vi "test write read channel.vi"() -> ()   [LabVIEW 2013]
doc: "This VI is an example of how to use subVIs from the BNC 500 series driver to programmatically configure multiple channels and the system timer (To). This VI initializes the pulse generator, gets the number of channels in the unit, configures individual channel(s), configures the system timer (To), initiate pulse generation, and then closes communications with the pulse generator. By default the VI DOES NOT stop pulse generation when exiting!!! Not all trigger and gate features are supported by all models covered by this driver. Selection of an unsupported function will generate a software error and the command is not sent to the hardware.\n\n\nNotes:\n1) The pulse generator keypad is returned to \"Local\" mode when this VI terminates in order to restore manual control to the user.\n2) VISA Version 3.3 or higher must be installed to use this instrument driver."
uses:
  <instrlib>/Berkeley Nucleonics 500 Series/Examples/Support/System Parameters.ctl
  <instrlib>/Berkeley Nucleonics 500 Series/Examples/Support/Channel Parameters.ctl
  <instrlib>/Berkeley Nucleonics 500 Series/Berkeley Nucleonics 500 Series.lvlib
panel:
  in  "read back":bool
  in  "Channel Parameters 2":T1={"Channel"=1, "Chan State"=TRUE, "Chan Sync Source"=0, "Chan Gate Logic"=enum."Disabled", "Chan Mode"=enum."Normal", "Chan Wait #"=40, "Chan Delay"=0.04, "Chan Width"=0.04, "Chan Burst #"=40, "Chan DC On"=40, "Chan DC Off"=40, "Chan Polarity"=FALSE, "Chan MUX Value"=-1, "Chan Level Out"=enum."Adjustable", "Chan Lev Adjust"=0.0, "Chan Gate Mode"=enum."Disabled"} {"Chan Sync Source" items=["System (To)", "Channel A", "Channel B", "Channel C", "Channel D", "Channel E", "Channel F", "Channel G", "Channel H"]; "Chan Width" format="%.3p"; "Chan Delay" format="%.3p"; "Chan Lev Adjust" format="%.3p"; "Channel" items=["Channel A"=1, "Channel B"=2, "Channel C"=3, "Channel D"=4, "Channel E"=5, "Channel F"=6, "Channel G"=7, "Channel H"=8]}
  out "Chan Parameters":T1={"Channel"=1, "Chan State"=TRUE, "Chan Sync Source"=0, "Chan Gate Logic"=enum."Disabled", "Chan Mode"=enum."Normal", "Chan Wait #"=-1, "Chan Delay"=nan, "Chan Width"=nan, "Chan Burst #"=-1, "Chan DC On"=-1, "Chan DC Off"=-1, "Chan Polarity"=FALSE, "Chan MUX Value"=-1, "Chan Level Out"=enum."TTL", "Chan Lev Adjust"=0.0, "Chan Gate Mode"=enum."Disabled"} {"Chan Sync Source" items=["System (To)", "Channel A", "Channel B", "Channel C", "Channel D", "Channel E", "Channel F", "Channel G", "Channel H"]; "Chan Width" format="%.3p"; "Chan Delay" format="%.3p"; "Chan Lev Adjust" format="%.3p"; "Channel" items=["Channel A"=1, "Channel B"=2, "Channel C"=3, "Channel D"=4, "Channel E"=5, "Channel F"=6, "Channel G"=7, "Channel H"=8]}
  out "System Parameters":T2={"Sys Period"=0.1, "Sys Mode"=enum."Normal", "Sys Burst #"=10, "Sys DC On"=10, "Sys DC Off"=10, "Sys State"=TRUE, "Sys Gate"=TRUE, "Sys Trig Edge"=TRUE, "Sys Ext Mode"=enum."Disabled", "Sys Trig Lev"=2.5, "Sys Gate Lev "=2.5, "Sys Gate Mode"=enum."Disabled"} {"Sys Gate Lev" format="%.4p"; "Sys Trig Lev" format="%.4p"; "Sys Period" format="%.6p"}
  in  "VISA resource":refnum<visa-resource-name>="COM1"
  in  "System Paramaters":T2={"Sys Period"=0.1, "Sys Mode"=enum."Normal", "Sys Burst #"=0, "Sys DC On"=10, "Sys DC Off"=20, "Sys State"=TRUE, "Sys Gate"=TRUE, "Sys Trig Edge"=TRUE, "Sys Ext Mode"=enum."Disabled", "Sys Trig Lev"=2.5, "Sys Gate Lev "=2.5, "Sys Gate Mode"=enum."Disabled"} {"Sys Gate Lev" format="%.4p"; "Sys Trig Lev" format="%.4p"; "Sys Period" format="%.6p"}
  # "500 Series\nPulse Generator\nExample Program"
  # "Notes:\n1.  The channel parameters \"Burst #\", \"DC On\", \"DC Off\", and \"Adjustable\" are only updated when operating in the corresponding mode.\n2.  The system parameters  \"Burst #\", \"DC On\", \"DC Off\", and \"Trig Level\"` are only updated when operating in the corresponding mode."
  # "Input"
  # "Normal\nSingle\nBurst"
  # "Burst"
  # "Duty Cycle"
  # "Output"
  # "Input"
  # "Normal\nSingle\nBurst"
  # "Burst"
  # "Duty Cycle"
  # "Output"
  # "Input"
  # "Triggered"
  # "Gated"
  # "Mode"
  # "Burst"
  # "Duty\nCycle"
  # "Input"
  # "Triggered"
  # "Gated"
  # "Mode"
  # "Burst"
  # "Duty\nCycle"
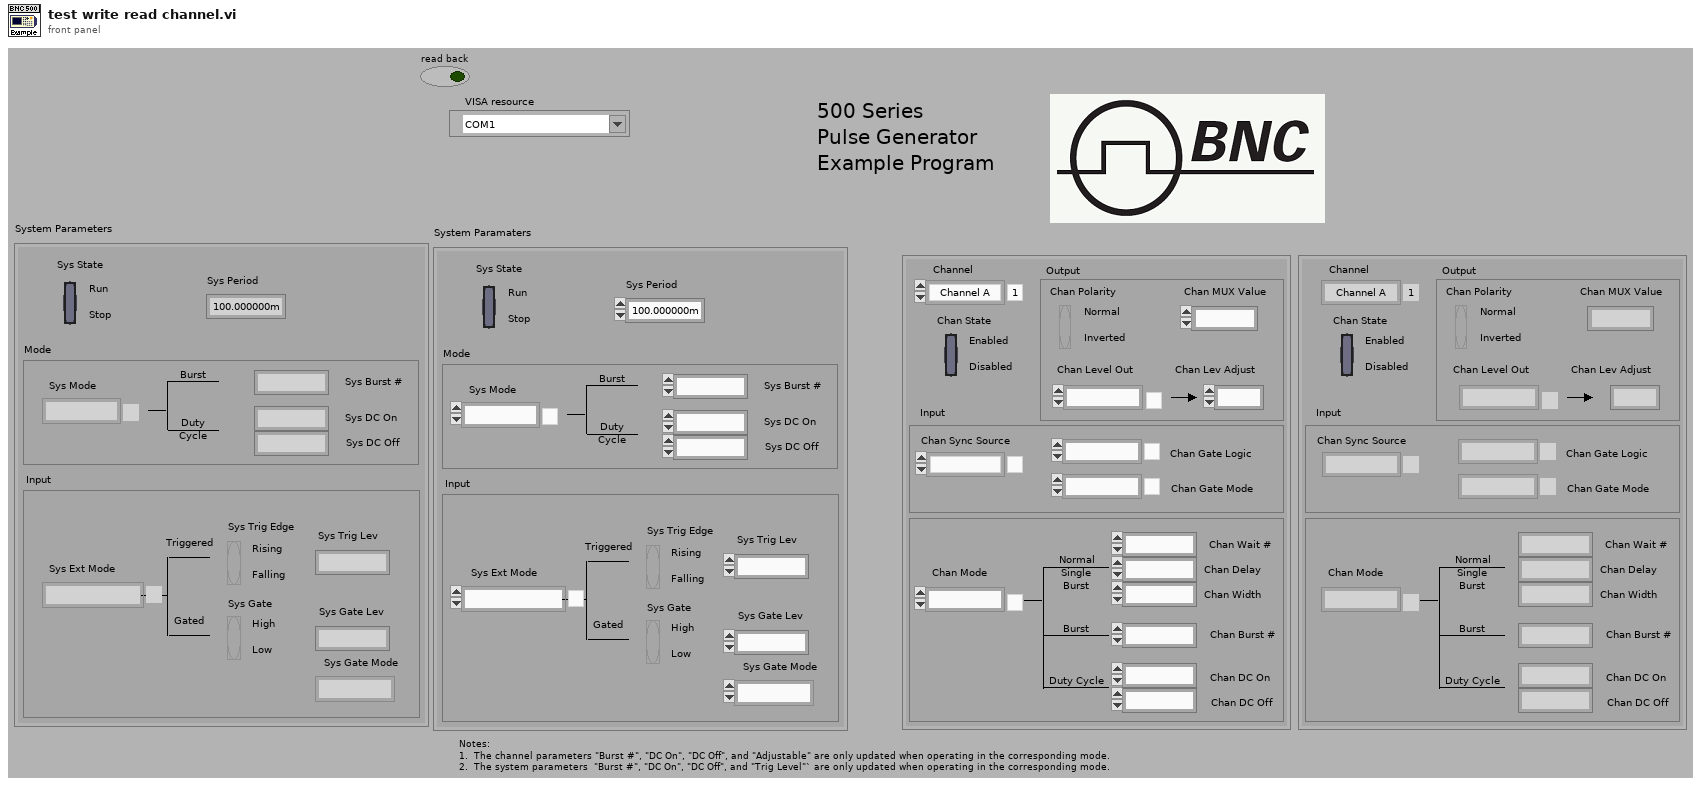
[diagram p1: front panel]
types:
  T1 = typedef "Channel Parameters.ctl" = cluster{"Channel":i32, "Chan State":bool, "Chan Sync Source":i32, "Chan Gate Logic":enum16{"Disabled", "Low", "High"}, "Chan Mode":enum16{"Normal", "Single", "Burst", "Duty Cycle"}, "Chan Wait #":i32, "Chan Delay":dbl, "Chan Width":dbl, "Chan Burst #":i32, "Chan DC On":i32, "Chan DC Off":i32, "Chan Polarity":bool, "Chan MUX Value":i32, "Chan Level Out":enum16{"TTL", "Adjustable", "35 Volt", "Optical"}, "Chan Lev Adjust":dbl, "Chan Gate Mode":enum16{"Disabled", "Pulse Inhibit", "Output Inhibit"}}
  T2 = typedef "System Parameters.ctl" = cluster{"Sys Period":dbl, "Sys Mode":enum16{"Normal", "Single", "Burst", "Duty Cycle"}, "Sys Burst #":i32, "Sys DC On":i32, "Sys DC Off":i32, "Sys State":bool, "Sys Gate":bool, "Sys Trig Edge":bool, "Sys Ext Mode":enum16{"Disabled", "Triggered", "Gated", "Triggered & Gated"}, "Sys Trig Lev":dbl, "Sys Gate Lev ":dbl, "Sys Gate Mode":enum16{"Disabled", "Pulse Inhibit", "Output Inhibit", "Channel"}}
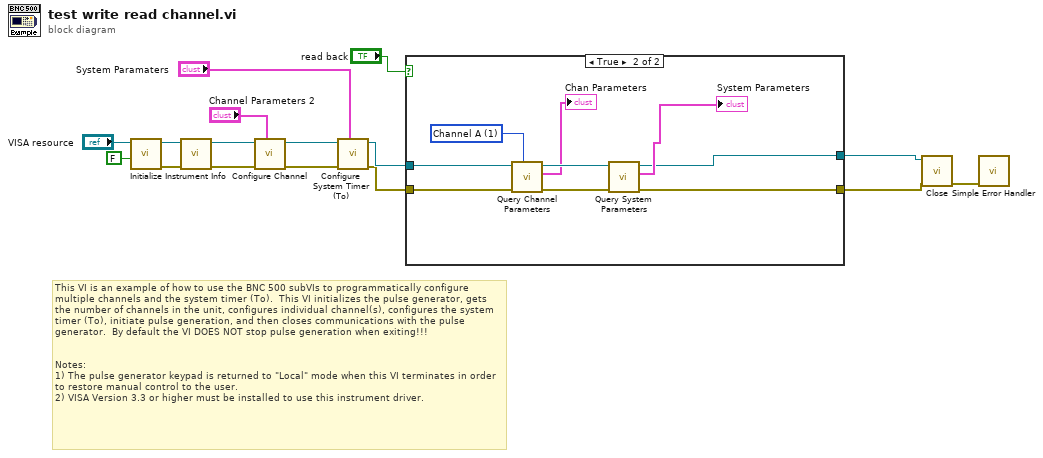
[diagram p0: block diagram]
diagram:
  # "This VI is an example of how to use the BNC 500 subVIs to programmatically configure multiple channels and the system timer (To).  This VI initializes the pulse generator, gets the number of channels in the unit, configures individual channel(s), configures the system timer (To), initiate pulse generation, and then closes communications with the pulse generator.  By default the VI DOES NOT stop pulse generation when exiting!!!\n\n\nNotes:\n1) The pulse generator keypad is returned to \"Local\" mode when this VI terminates in order to restore manual control to the user.\n2) VISA Version 3.3 or higher must be installed to use this instrument driver."
  n1 = call <instrlib>:"Initialize.vi"("Reset? (T: Yes)"=FALSE, "VISA resource name"="VISA resource") -> ("error out"=w11:errorcluster, "VISA resource name out"=w12:refnum<visa-resource-name>)  [unwired: 8 in]
  n2 = call <instrlib>:"Instrument Info.vi"("error in (no error)"=w11, "VISA resource name"=w12) -> ("error out"=w9:errorcluster, "VISA resource name out"=w13:refnum<visa-resource-name>)  [unwired: 6 in, 2 out]
  n3 = call <instrlib>:"Configure Channel.vi"("Chan Parameters"="Channel Parameters 2", "error in (no error)"=w9, "VISA resource name"=w13) -> ("error out"=w10:errorcluster, "VISA resource name out"=w16:refnum<visa-resource-name>)  [unwired: 7 in]
  n4 = call <instrlib>:"Configure System Timer (To).vi"("System Parameters"="System Paramaters", "error in (no error)"=w10, "VISA resource name"=w16) -> ("error out"=w5:errorcluster, "VISA resource name out"=w6:refnum<visa-resource-name>)  [unwired: 7 in]
  n5 = case shown="True" "read back" {
    tunnel: w6 -> [w18 w24]
    tunnel: w5 -> [w17 w23]
    tunnel: [w18 w22] -> w4
    tunnel: [w17 w21] -> w3
    frame False {
    }
    frame True {
      w19 = 1 items=["Channel A"=1, "Channel B"=2, "Channel C"=3, "Channel D"=4, "Channel E"=5, "Channel F"=6, "Channel G"=7, "Channel H"=8] ("Channel (1:Chan A)")
      n6 = call <instrlib>:"Query Channel Parameters.vi"("Channel (1:Chan A)"=w19, "error in (no error)"=w23, "VISA resource name"=w24) -> ("error out"=w26:errorcluster, "Chan Parameters"=→"Chan Parameters":T1, "VISA resource name out"=w27:refnum<visa-resource-name>)  [unwired: 6 in]
      n7 = call <instrlib>:"Query System Parameters.vi"("error in (no error)"=w26, "VISA resource name"=w27) -> ("error out"=w21:errorcluster, "System Parameters"=→"System Parameters":T2, "VISA resource name out"=w22:refnum<visa-resource-name>)  [unwired: 7 in]
    }
  }
  n8 = call <instrlib>:"Close.vi"("error in (no error)"=w3, "VISA resource name"=w4) -> ("error out"=w8:errorcluster)  [unwired: 9 in]
  n9 = call <vilib>:"Simple Error Handler.vi"("error in (no error)"=w8) -> ()  [unwired: 4 in, 5 out]
